vi "Write Array Ini.vi"(8 "error in (no error)":errorcluster, 10 "Write_key":string[](array[string]), 11 "Section":string) -> (0 "error out":errorcluster)   [LabVIEW 2020]
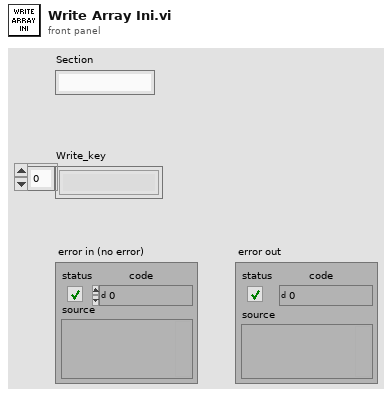
[diagram p1: front panel]
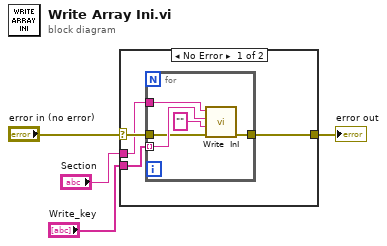
[diagram p0: block diagram]
diagram:
  n1 = case shown="No Error" "error in (no error)" {
    selector: "error in (no error)" -> [w7 w14]
    tunnel: "Write_key" -> [w8 _]
    tunnel: "Section" -> [w6 _]
    tunnel: [w5 w14] -> w1
    frame No Error {
      n2 = for {
        tunnel: w8 -> [w12] mode=indexing
        tunnel: w7 -> [w10]
        tunnel: w6 -> [w13]
        tunnel: [w9] -> w5
        n3 = call "Write  InI.vi"("error in (no error)"=w10, "value"="", "key"=w12, "section"=w13) -> ("error out"=w9:errorcluster)  [unwired: 6 in, 1 out]
      }
    }
    frame Error {
    }
  }
  "error out" <- w1
